vi "VPA QC Update Volume Cal Numbers.vi"(9 "DAQ Ref Cluster":T1, 10 "Cyl. Vol. Calibration Data":T3 {"Average Difference" format="%#.5g"; "Volume to Flow" step=0.1 format="%#_4g"; "Average" format="%#.5g"; "% Difference 3" format="%#.5g"; "% Difference 2" format="%#.5f"; "% Difference 1" format="%#.5f"}) -> ()   [LabVIEW 2013]
uses:
  VPA QC Vol Cal Data Cluster.ctl
  Controls/VPA QC DAQ Ref Cluster.ctl
  Controls/VPA QC Scale Communication Settings DVR.ctl
  Controls/VPA QC Scale Communication Settings.ctl
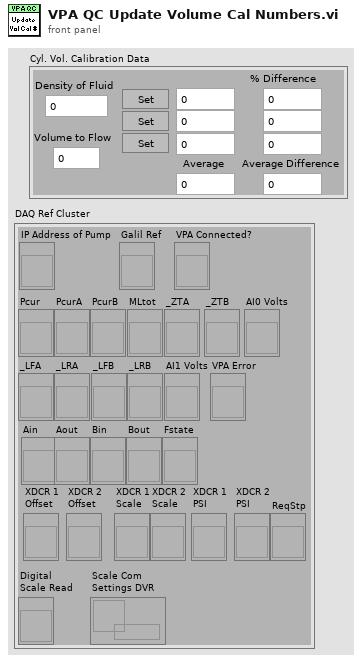
[diagram p1: front panel]
types:
  T1 = typedef "VPA QC DAQ Ref Cluster.ctl" = cluster{"IP Address of Pump":refnum<vi>, "Galil Ref":refnum<vi>, "VPA Connected?":refnum<vi>, "Pcur":refnum<vi>, "PcurA":refnum<vi>, "PcurB":refnum<vi>, "MLtot":refnum<vi>, "_LFA":refnum<vi>, "_LRA":refnum<vi>, "_LFB":refnum<vi>, "_LRB":refnum<vi>, "_ZTA":refnum<vi>, "_ZTB":refnum<vi>, "AI0 Volts":refnum<vi>, "AI1 Volts":refnum<vi>, "VPA Error":refnum<vi>, "Ain":refnum<vi>, "Aout":refnum<vi>, "Bin":refnum<vi>, "Bout":refnum<vi>, "Fstate":refnum<vi>, "XDCR 1\nOffset":refnum<vi>, "XDCR 2 \nOffset":refnum<vi>, "XDCR 1\nScale":refnum<vi>, "XDCR 2\nScale":refnum<vi>, "XDCR 1\nPSI":refnum<vi>, "XDCR 2\nPSI":refnum<vi>, "ReqStp":refnum<vi>, "Digital \nScale Read":refnum<vi>, "Scale Com\nSettings DVR":T2}
  T2 = typedef "VPA QC Scale Communication Settings DVR.ctl" = refnum<data-value>
  T3 = typedef "VPA QC Vol Cal Data Cluster.ctl" = cluster{"Volume Measured 1":dbl, "Volume Measured 2":dbl, "Volume Measured 3":dbl, "% Difference 1":dbl, "% Difference 2":dbl, "% Difference 3":dbl, "Average":dbl, "Volume to Flow":dbl, "Density of Fluid":dbl, "Set Vol 1":bool, "Set Vol 2":bool, "Set Vol 3":bool, "Average Difference":dbl}
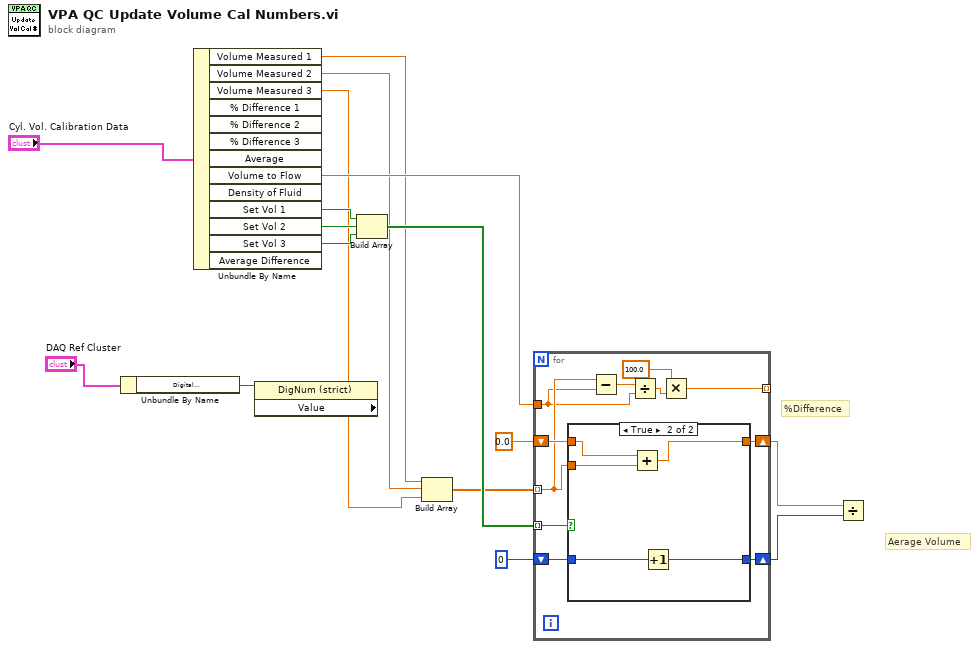
[diagram p0: block diagram]
diagram:
  # "%Difference"
  # "Aerage Volume"
  n1 = Unbundle By Name("DAQ Ref Cluster") -> ("Digital \nScale Read"=w11:refnum<vi>)
  n2 = Unbundle By Name("Cyl. Vol. Calibration Data") -> ("Volume Measured 1"=w4:dbl, "Volume Measured 2"=w3:dbl, "Volume Measured 3"=w2:dbl, "Volume to Flow"=w5:dbl, "Set Vol 1"=w16:bool, "Set Vol 2"=w15:bool, "Set Vol 3"=w14:bool)  [unwired: 6 out]
  n3 = property class="DigNum (strict)" props=["Value"](reference=w11) -> ()  [unwired: 1 in, 3 out]
  n4 = Build Array(w16, w15, w14) -> (w10:bool[])
  n5 = Build Array(w4, w3, w2) -> (w1:dbl[])
  n6 = for {
    tunnel: w10 -> [w27] mode=indexing
    shift-right: [w25] -> w7
    shift-left: 0.0 -> [w26]
    shift-right: [w23] -> w6
    shift-left: u8 0 -> [w24]
    tunnel: w5 -> [w18]
    tunnel: w1 -> [w19] mode=indexing
    tunnel: [w17] -> _ mode=indexing
    n7 = case shown="True" w27 {
      tunnel: w26 -> [w29 w34]
      tunnel: w19 -> [_ w30]
      tunnel: [w29 w33] -> w25
      tunnel: [w28 w31] -> w23
      tunnel: w24 -> [w28 w32]
      frame False {
      }
      frame True {
        n8 = Add(x=w34, y=w30) -> (x+y=w33:dbl)
        n9 = Increment(x=w32) -> (x+1=w31:u8)
      }
    }
    n10 = Subtract(x=w19, y=w18) -> (x-y=w22:dbl)
    n11 = Divide(x=w22, y=w18) -> (x/y=w21:dbl)
    n12 = Multiply(x=100.0, y=w21) -> (x*y=w17:dbl)
  }
  n13 = Divide(x=w7, y=w6) -> ()  [unwired: 1 out]
